vi "PLC test.vi"() -> ()   [LabVIEW 2017]
uses:
  <vilib>/DATA AHEAD/SP7/typedefs/PLC Type.ctl
  <vilib>/DATA AHEAD/SP7/functions/read/read Dint array.vi
  <vilib>/DATA AHEAD/SP7/functions/read/read String.vi
  <vilib>/DATA AHEAD/SP7/SP7.lvlib
panel:
  in  "Data Block No":u16=7
  out "2nd block":errorcluster
  in  "Items # [byte] 2":u16=1 caption="Items count [byte]"
  in  "String length in DB":u16=50
  in  "Item offset [byte] 2":u32=24 caption="Item offset [byte]"
  in  "Block 2":bool
  in  "Block 1":bool
  in  "Item offset [byte]":u32
  in  "No. of Items[byte]":u16=1
  in  "Data Block #":u16=7
  in  "IP address":string="192.168.0.80"
  out "1st block":errorcluster
  out "DINT read":i32[](array[numeric])
  out "STRING result Array":string[](array[string])
  out "PLC Connection Error Status":errorcluster
  in  "stop":bool
  # "String Read Array"
  # "Dint Read Array"
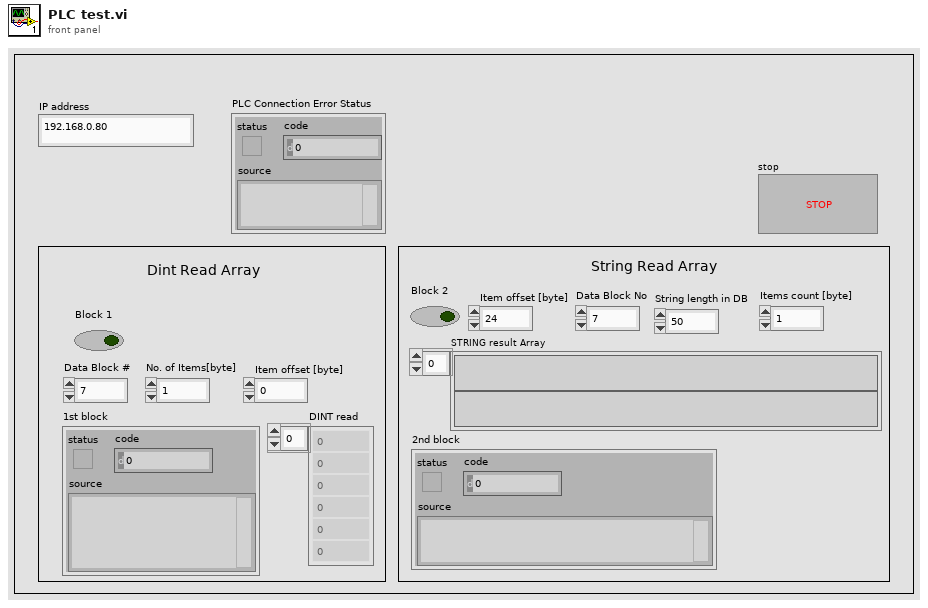
[diagram p1: front panel]
types:
  T1 = typedef "SP7.lvlib/PLC Type.ctl" = enum16{"S7 200", "S7 300/400", "S7 1200", "S7 1500", "LOGO!8"}
  T2 = typedef "SP7.lvlib/S7 Connection.ctl" = cluster{"TCP Connection Ref":refnum<k5>, "IP address":string, "timeout ms":i32, "Connected?":bool, "PLC Type":T1, "Rack S7 400":u8, "Slot S7 400":u8, "PDU Size":u16, "connection semaphore":T3}
  T3 = typedef "Semaphore RefNum" = refnum<k1>
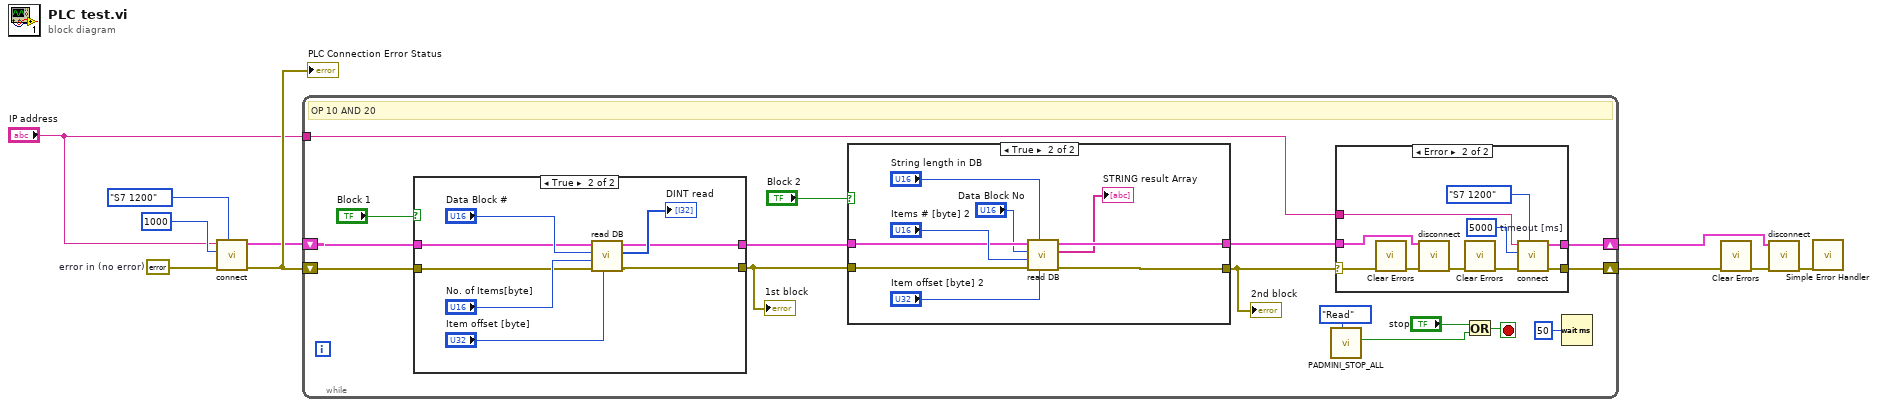
[diagram p0: block diagram]
diagram:
  w2 = errorcluster {"status"=FALSE, "code"=0, "source"=""}  # error in (no error)
  n1 = call <vilib>:"connect.vi"("PLC Type"=PLC_Type."S7 1200" ("PLC Type 2"), "error in (no error)"=w2, "timeout [ms]"=1000, "IP address"="IP address") -> ("error out"=w7:errorcluster, "S7 Connection out"=w6:T2)  [unwired: 6 in]
  "PLC Connection Error Status" <- w7
  n2 = while {
    shift-right: [w18] -> w4
    shift-left: w6 -> [w26]
    shift-right: [w19] -> w10
    shift-left: w7 -> [w25]
    tunnel: "IP address" -> [w17]
    stop <- w20 stop-if-true
    # "OP 10 AND 20"
    n3 = case shown="True" "Block 1" {
      tunnel: [w40 w45] -> w15
      tunnel: w26 -> [w40 w44]
      tunnel: w25 -> [w39 w43]
      tunnel: [w39 w42] -> w12
      frame False {
      }
      frame True {
        n4 = call-poly <vilib>:"read DB.vi"("Item offset [byte]"="Item offset [byte]", "error in (no error)"=w43, "items #"="No. of Items[byte]", "Data Block #"="Data Block #", "S7 Connection in"=w44) -> ("error out"=w42:errorcluster, "DINT result array"=→"DINT read":i32[], "S7 Connection out"=w45:T2)  [unwired: 4 in]
      }
    }
    "1st block" <- w12
    n5 = case shown="True" "Block 2" {
      tunnel: w12 -> [w50 w56]
      tunnel: [w50 w53] -> w11
      tunnel: [w49 w54] -> w16
      tunnel: w15 -> [w49 w55]
      frame False {
      }
      frame True {
        n6 = call-poly <vilib>:"read DB.vi"("Item offset [byte]"="Item offset [byte] 2", "String length reserved in DB (default=254)"="String length in DB", "error in (no error)"=w56, "items #"="Items # [byte] 2", "Data Block #"="Data Block No", "S7 Connection in"=w55) -> ("error out"=w53:errorcluster, "STRING result Array"=→"STRING result Array":string[], "S7 Connection out"=w54:T2)  [unwired: 2 in, 1 out]
      }
    }
    "2nd block" <- w11
    n7 = call "PADMINI_STOP_ALL.vi"("Enum"=enum16{"Read", "Write"}."Read") -> ("Boolean 2"=w22:bool)  [unwired: 9 in, 1 out]
    n8 = case shown="Error" w11 {
      selector: w11 -> [w28 w37]
      tunnel: [w27 w30] -> w18
      tunnel: [w28 w35] -> w19
      tunnel: w16 -> [w27 w32]
      tunnel: w17 -> [_ w31]
      frame No Error {
      }
      frame Error {
        w29 = 5000  # timeout [ms]
        n9 = call <vilib>:"Clear Errors.vi"("error in (no error)"=w37) -> ("error out"=w38:errorcluster)  [unwired: 5 in, 1 out]
        n10 = call <vilib>:"disconnect.vi"("error in (no error)"=w38, "S7 Connection in"=w32) -> ("error out"=w36:errorcluster)  [unwired: 8 in, 1 out]
        n11 = call <vilib>:"Clear Errors.vi"("error in (no error)"=w36) -> ("error out"=w34:errorcluster)  [unwired: 5 in, 1 out]
        n12 = call <vilib>:"connect.vi"("PLC Type"=PLC_Type."S7 1200" ("PLC Type 2"), "error in (no error)"=w34, "timeout [ms]"=w29, "IP address"=w31) -> ("error out"=w35:errorcluster, "S7 Connection out"=w30:T2)  [unwired: 6 in]
      }
    }
    n13 = Or(x="stop", y=w22) -> (x .or. y?=w20:bool)
    n14 = Wait (ms)(milliseconds to wait=u32 50) -> ()  [unwired: 1 out]
  }
  n15 = call <vilib>:"Clear Errors.vi"("error in (no error)"=w10) -> ("error out"=w5:errorcluster)  [unwired: 5 in, 1 out]
  n16 = call <vilib>:"disconnect.vi"("error in (no error)"=w5, "S7 Connection in"=w4) -> ("error out"=w1:errorcluster)  [unwired: 8 in, 1 out]
  n17 = call <vilib>:"Simple Error Handler.vi"("error in (no error)"=w1) -> ()  [unwired: 4 in, 5 out]
